vi "Ease Panel.vi"(8 "error in (no error)":errorcluster) -> (0 "error out":errorcluster)   [LabVIEW 2011, in "Sliding Menu Library.lvlib"]
uses:
  Sliding Menu Library.lvlib
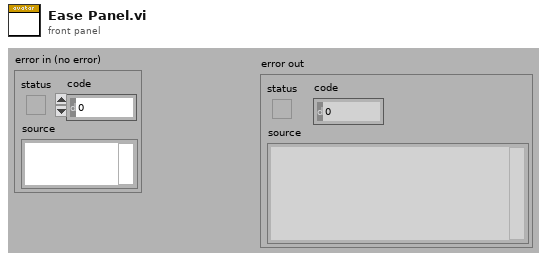
[diagram p1: front panel]
types:
  T1 = typedef "Sliding Menu Library.lvlib/User Interface Type Definitions.ctl" = cluster{"This VI":refnum<vi>, "User Interace Plugin":refnum<vi>, "Title String":refnum<vi>, "Message Display":refnum<vi>, "Array of Menu Button References":refnum<vi>[], "config file refnum":T2}
  T2 = typedef "NI_LVConfig.lvlib/Config Data RefNum.ctl" = refnum<k1>
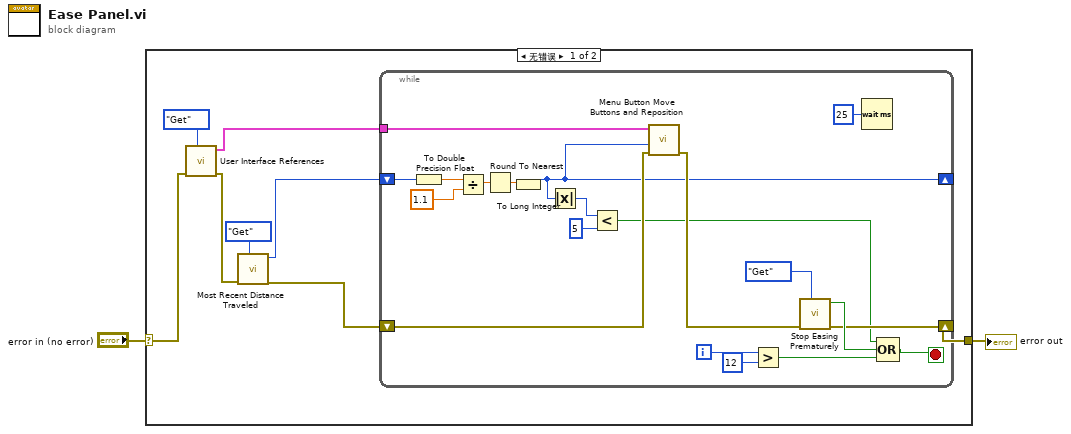
[diagram p0: block diagram]
diagram:
  n1 = case shown="无错误" "error in (no error)" {
    selector: "error in (no error)" -> [w5 w31]
    tunnel: [w10 w31] -> w2
    frame No Error {
      n2 = call "User Interface References.vi"("Set or Get Value"=enum16{"Set", "Get"}."Get", "error in"=w5) -> ("error out"=w4:errorcluster, "User Interface References 2"=w6:T1)  [unwired: 8 in]
      n3 = call "Most Recent Distance Traveled.vi"("Set or Get Value"=enum16{"Set", "Get"}."Get", "error in"=w4) -> ("error out"=w7:errorcluster, "Saved Distance"=w8:i32)  [unwired: 8 in]
      n4 = while {
        shift-right: [w17] -> w10
        shift-left: w7 -> [w29]
        shift-right: [w14] -> _
        shift-left: w8 -> [w28]
        tunnel: w6 -> [w30]
        i -> [w24]
        stop <- w22 stop-if-true
        n5 = To Double Precision Float(number=w28) -> (double precision float=w27:dbl)
        n6 = Divide(x=w27, y=1.1) -> (x/y=w11:dbl)
        n7 = Round To Nearest(number=w11) -> (nearest integer value=w12:dbl)
        n8 = To Long Integer(number=w12) -> (32bit integer=w14:i32)
        n9 = Absolute Value(x=w14) -> (abs(x)=w13:i32)
        n10 = Less?(x=w13, y=5) -> (x < y?=w15:bool)
        n11 = call "Menu Button Move Buttons and Reposition.vi"("error in (no error)"=w29, "Distance"=w14, 11:w30) -> ("error out"=w18:errorcluster)  [unwired: 6 in, 2 out]
        n12 = Greater?(x=w24, y=12) -> (0:w21:bool)
        n13 = call "Stop Easing Prematurely.vi"("Set or Get Value"=enum16{"Set", "Get"}."Get", "error in"=w18) -> ("error out"=w17:errorcluster, "Stop?"=w19:bool)  [unwired: 8 in]
        n14 = Wait (ms)(milliseconds to wait=u32 25) -> ()  [unwired: 1 out]
        n15 = Compound Arithmetic op=OR(w15, w19, w21) -> (w22:bool)
      }
    }
    frame Error {
    }
  }
  "error out" <- w2
